vi "registerCommand.vi"(8 "error in (no error)":errorcluster, 10 "registeredCommands":string[](array[string]), 11 "tcpServer in":refnum<class "TcpServer.lvclass">) -> (0 "error out":errorcluster, 3 "tcpServer out":refnum<class "TcpServer.lvclass">)   [LabVIEW 2018, in "TcpServer.lvclass"]
doc: "Inform the TCP Server which commands are registered and allowed to be used by LabVIEW Component."
uses:
  TcpServer.lvclass
  TcpServer.lvclass/TcpServer.ctl
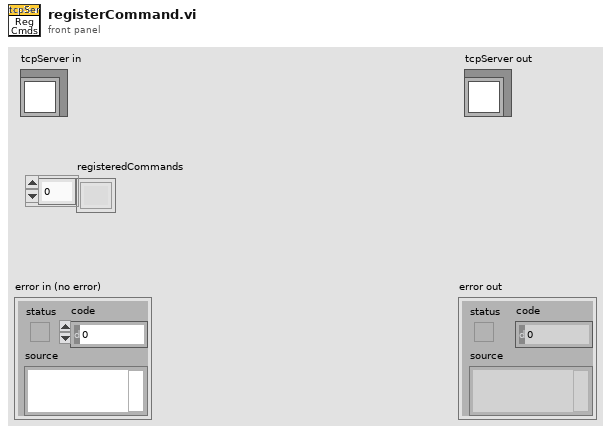
[diagram p1: front panel]
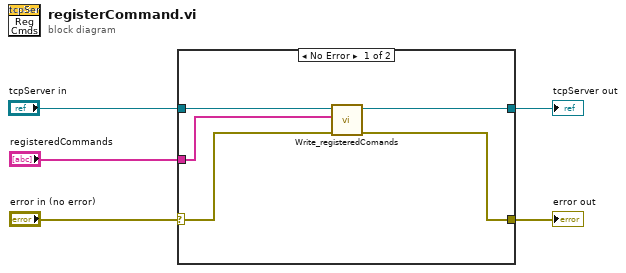
[diagram p0: block diagram]
diagram:
  n1 = case shown="No Error" "error in (no error)" {
    selector: "error in (no error)" -> [w7 w12]
    tunnel: [w6 w12] -> w4
    tunnel: [w9 w11] -> w2
    tunnel: "tcpServer in" -> [w10 w11]
    tunnel: "registeredCommands" -> [w8 _]
    frame No Error {
      n2 = call "Write_registeredComands.vi"("error in (no error)"=w7, "registeredCommands"=w8, "TcpServer in"=w10) -> ("error out"=w6:errorcluster, "TcpServer out"=w9:refnum<class "TcpServer.lvclass">)  [unwired: 7 in]
    }
    frame Error {
    }
  }
  "error out" <- w4
  "tcpServer out" <- w2
